vi "TEST.vi"() -> ()   [LabVIEW 2013]
uses:
  <vilib>/Instr/_visa.llb/VISA Configure Serial Port (Instr).vi
panel:
  out "Axis":string
  in  "포트":u16=50
  in  "IP":string="127.0.0.1"
  in  "RDelay":u32
  out "불리언":bool
  out "Write":string
  in  "Motor R":u32(slide)=128 scale=0.0..255.0
  in  "Motor M":u32(slide)=128 scale=0.0..255.0
  in  "Motor L":u32(slide)=128 scale=0.0..255.0
  in  "정지 버튼":bool
  in  "Delay":u32=500
  in  "RUN":bool
  out "WORK":i32
  in  "VISA resource name":refnum<visa-resource-name>="COM3"
  in  "Serial Settings":T1={"baud rate"=9600, "data bits"=8, "parity"=enum."None", "stop bits"=10, "flow control"=0} {"flow control" items=["None"=0, "XON/XOFF"=1, "RTS/CTS"=2, "DTR/DSR"=4]; "stop bits" items=["1.0"=10, "1.5"=15, "2.0"=20]; "data bits" min=5 max=8 step=1; "baud rate" items=["75"=75, "110"=110, "134"=134, "150"=150, "300"=300, "600"=600, "1200"=1200, "1800"=1800, "2400"=2400, "4800"=4800, "7200"=7200, "9600"=9600, "14400"=14400, "19200"=19200, "28800"=28800, "38400"=38400, "56000"=56000, "57600"=57600, "115200"=115200, "128000"=128000, "230400"=230400]}
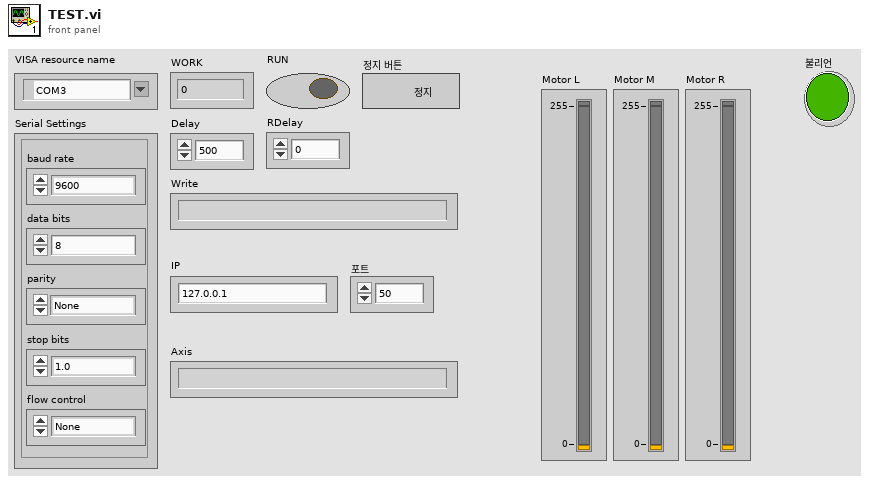
[diagram p1: front panel]
types:
  T1 = cluster{"baud rate":u32, "data bits":u16, "parity":enum16{"None", "Odd", "Even", "Mark", "Space"}, "stop bits":u16, "flow control":u16}
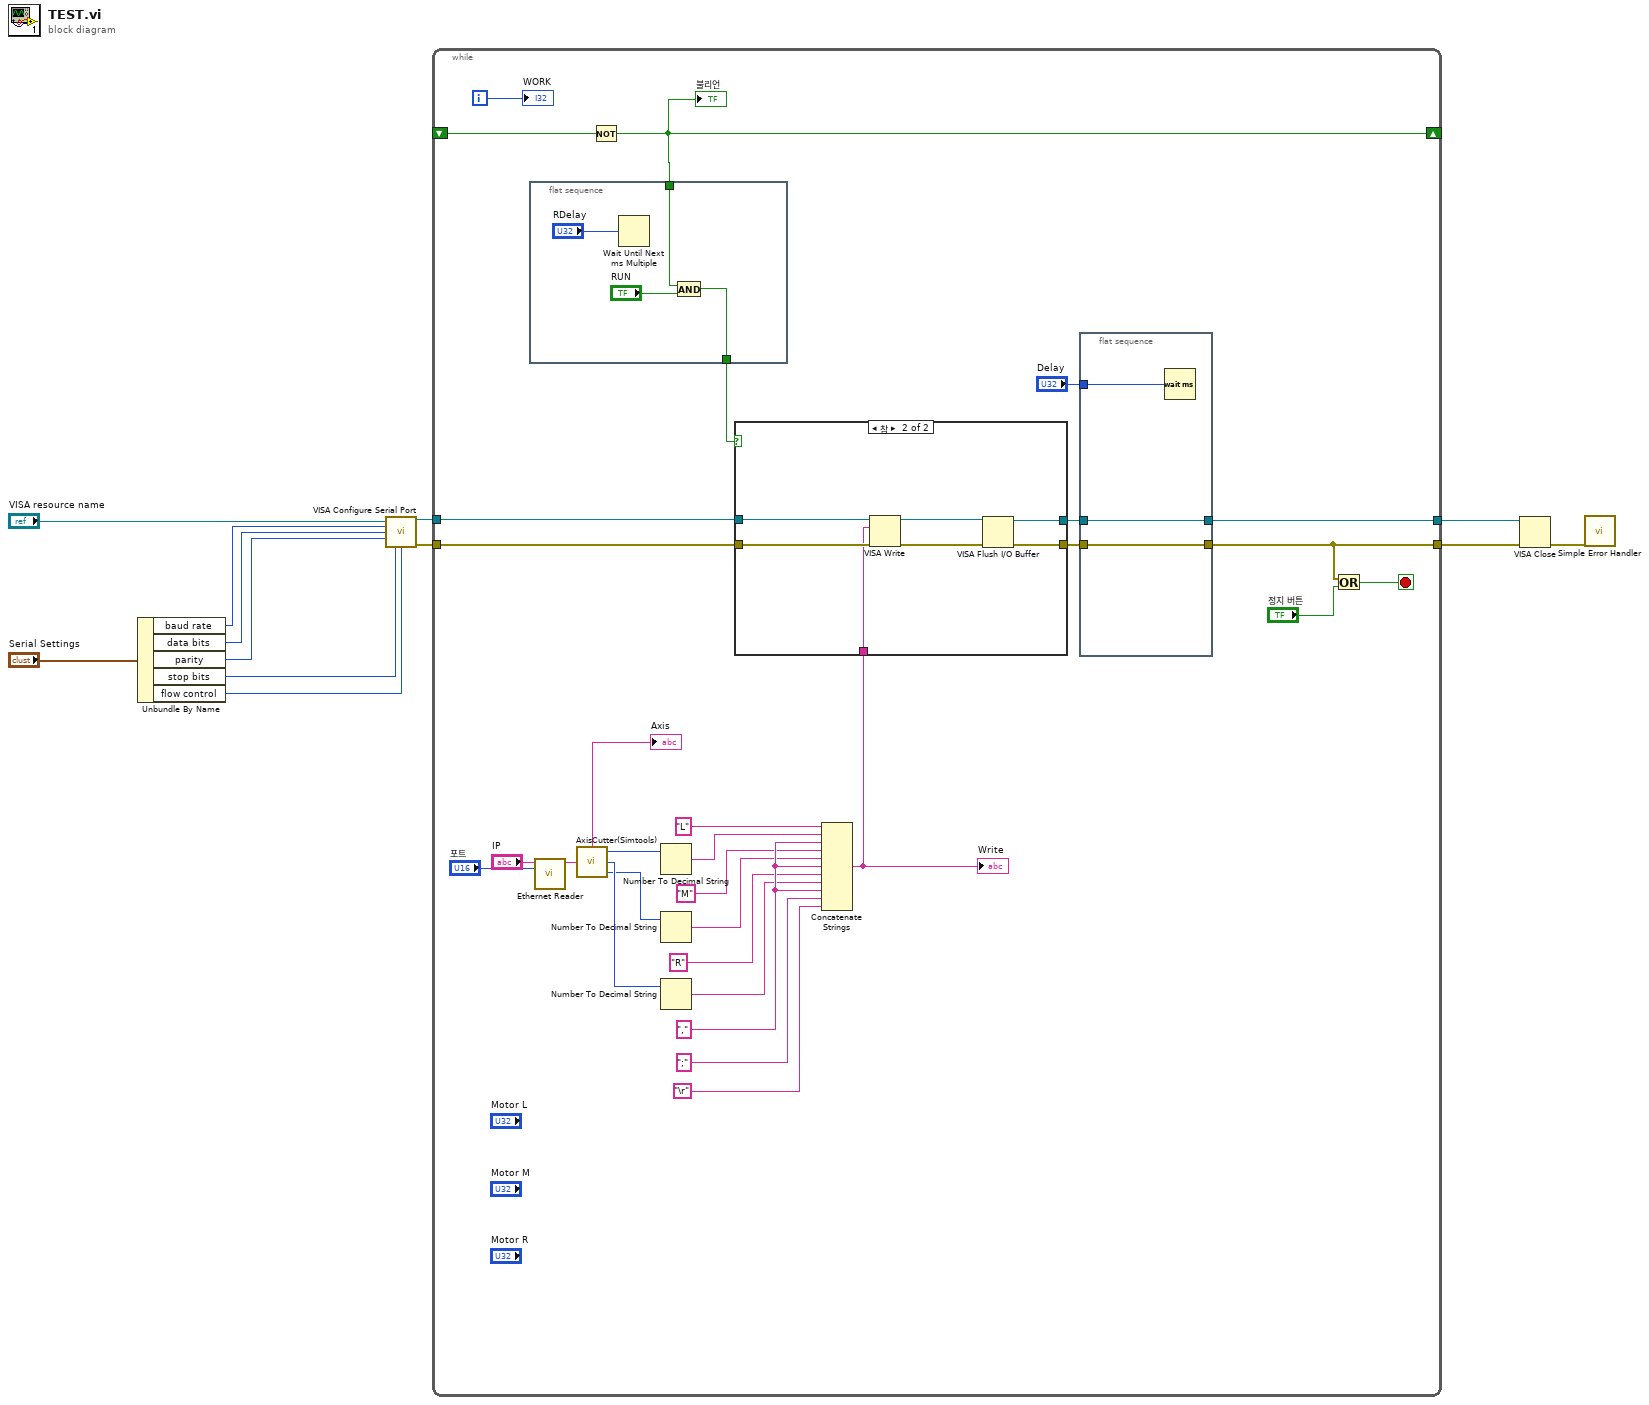
[diagram p0: block diagram]
diagram:
  n1 = Unbundle By Name("Serial Settings") -> ("baud rate"=w5:u32, "data bits"=w4:u16, "parity"=w3:enum16{"None", "Odd", "Even", "Mark", "Space"}, "stop bits"=w2:u16, "flow control"=w1:u16)
  n2 = call-poly "VISA Configure Serial Port"("VISA resource name"="VISA resource name", "baud rate (9600)"=w5, "data bits (8)"=w4, "parity (0:none)"=w3, "stop bits (10: 1 bit)"=w2, "flow control (0:none)"=w1) -> ("VISA resource name out"=w12:refnum<visa-resource-name>, "error out"=w11:errorcluster)  [unwired: 8 in]
  n3 = while {
    tunnel: w12 -> [w42]
    tunnel: w11 -> [w41]
    tunnel: [w36] -> w9
    tunnel: [w25] -> w8
    shift-right: [w21] -> _
    shift-left: _ -> [w23]
    i -> [w37]
    stop <- w26 stop-if-true
    w33 = ","
    n4 = flat-sequence {
      tunnel: [w46] -> w22
      tunnel: w21 -> [w45]
      frame #0 {
        n5 = Wait Until Next ms Multiple(millisecond multiple="RDelay") -> ()  [unwired: 1 out]
        n6 = And(x=w45, y="RUN") -> (x .and. y?=w46:bool)
      }
    }
    n7 = call "Ethernet Reader.vi"("IP"="IP", "포트"="포트") -> ("Axis"=w18:string)  [unwired: 6 in, 1 out]
    n8 = call "AxisCutter(Simtools).vi"("수신"=w18) -> ("Axis"=→"Axis":string, "L"=w16:i32, "R"=w15:i32, "M"=w14:i32)
    n9 = Not(x=w23) -> (.not. x?=w21:bool)
    "불리언" <- w21
    n10 = Number To Decimal String(number=w16) -> (decimal integer string=w34:string)  [unwired: 1 in]
    n11 = Number To Decimal String(number=w14) -> (decimal integer string=w31:string)  [unwired: 1 in]
    n12 = Number To Decimal String(number=w15) -> (decimal integer string=w29:string)  [unwired: 1 in]
    n13 = Concatenate Strings("L", w34, w33, "M", w31, w33, "R", w29, w33, ";", "\r") -> (w17:string)
    "Write" <- w17
    n14 = case shown="참" w22 {
      tunnel: w42 -> [w51 w58]
      tunnel: w41 -> [w50 w57]
      tunnel: [w51 w54] -> w40
      tunnel: [w50 w53] -> w39
      tunnel: w17 -> [_ w52]
      frame False {
      }
      frame True {
        n15 = VISA Write(VISA resource name=w58, write buffer=w52, error in (no error)=w57) -> (VISA resource name out=w56:refnum<visa-resource-name>, error out=w55:errorcluster)  [unwired: 1 out]
        n16 = VISA Flush I/O Buffer(VISA resource name=w56, error in (no error)=w55) -> (VISA resource name out=w54:refnum<visa-resource-name>, error out=w53:errorcluster)  [unwired: 1 in]
      }
    }
    n17 = flat-sequence {
      tunnel: w40 -> [w48]
      tunnel: w39 -> [w47]
      tunnel: "Delay" -> [w49]
      tunnel: [w48] -> w36
      tunnel: [w47] -> w25
      frame #0 {
        n18 = Wait (ms)(milliseconds to wait=w49) -> ()  [unwired: 1 out]
      }
    }
    n19 = Or(x=w25, y="정지 버튼") -> (x .or. y?=w26:bool)
    "WORK" <- w37
  }
  n20 = VISA Close(VISA resource name=w9, error in (no error)=w8) -> (error out=w10:errorcluster)
  n21 = call <vilib>:"Simple Error Handler.vi"("error in (no error)"=w10) -> ()  [unwired: 1 in, 8 out]
